vi "Exemple_Preprocessing_LabelEncoder.vi"() -> ()   [LabVIEW 2020]
uses:
  Objet/6 - Datasets Transformation/6.3 - Processing Data/LabelEncoder/LabelEncoder.lvclass
panel:
  in  "y":string[][](array[string])=[["paris"], ["paris"], ["tokyo"], ["amsterdam"]]
  out "Data":T1
  out "error out":errorcluster
  in  "error in":errorcluster caption="entrée d'erreur"
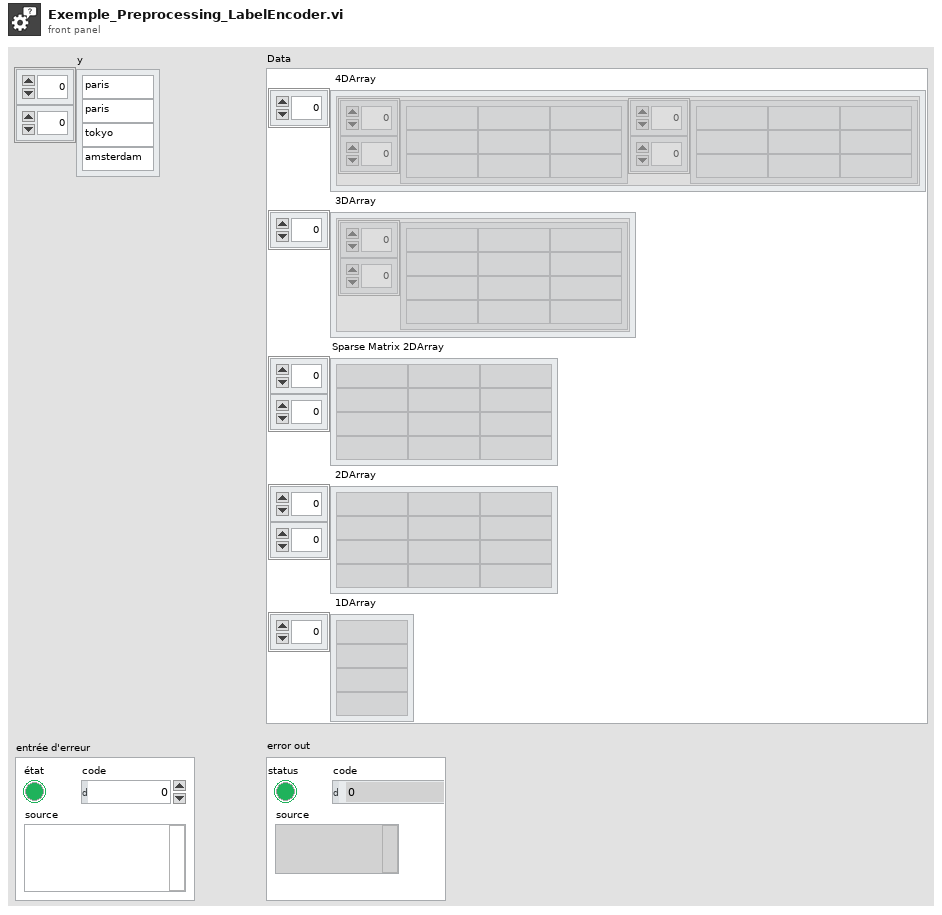
[diagram p1: front panel]
types:
  T1 = cluster{" 4DArray":cluster{"1":string[][], "2":string[][]}[], " 3DArray":cluster{"Tableau":string[][]}[], "Sparse Matrix 2DArray":string[][], " 2DArray":string[][], " 1DArray":string[]}
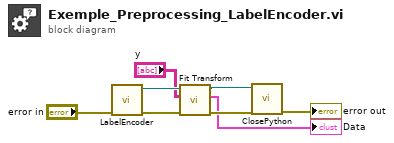
[diagram p0: block diagram]
diagram:
  n1 = call "LabelEncoder.vi"("error in (no error)"="error in") -> ("error out"=w5:errorcluster, "LabelEncoder.lvclass"=w7:refnum<class "LabelEncoder.lvclass">)  [unwired: 9 in]
  n2 = call-dynamic "Fit Transform.vi"("error in (no error)"=w5, "y"="y", "LabelEncoder.lvclass"=w7) -> ("error out"=w3:errorcluster, "Data"=→"Data":T1, "LabelEncoder.lvclass"=w4:refnum<class "LabelEncoder.lvclass">)  [unwired: 6 in]
  n3 = call-dynamic "ClosePython.vi"("error in (no error)"=w3, "Scikit-learn en entrée"=w4) -> ("error out"=→"error out":errorcluster)  [unwired: 8 in, 1 out]
